vi "log analysis_gps.vi"() -> ()   [LabVIEW 2019] (continued)
76.149993\t101.748821\t8.130800\t-0.795731\t0.628381\t-123.867001\t0.539000\t-0.099000\n\t\n15:49:11.8\tlog_raw\tgps_raw\t#INSPVAXA,USB3,0,49.0,FINESTEERING,2107,283769.800,02000000,471d,15824;INS_ALIGNMENT_COMPLETE,INS_RTKFIXED,37.37104525737,126.72169313095,8.1331,22.3000,-0.3548,-0.2589,0.0390,-0.749813070,0.572311932,213.822472384,0.4366,0.3042,0.5948,0.1140,0.0941,0.0845,0.0971,0.1011,5.0877,0f000001,0*7155f04b\n\tsystem status\tnormal 2 27.800000 0 0\trobot status\t76.002525\t101.557319\t8.133100\t-0.749813\t0.572312\t-123.822472\t0.465000\t0.046000\n\t\n15:49:12.3\tlog_raw\tgps_raw\t#DUALANTENNAHEADINGA,USB3,0,51.5,FINESTEERING,2107,283770.300,02000000,d426,15824;INSUFFICIENT_OBS,NONE,-1.000000000,0.000000000,0.000000000,0.0,0.000000000,0.000000000,\"631T\",11,2,2,2,04,00,20,00*c0be82b5\n\tsystem status\tnormal 2 27.700000 0 0\trobot status\t75.860019\t101.367468\t8.133800\t-0.793741\t0.557880\t-123.760851\t0.448000\t0.089000\n\t\n15:49:12.8\tlog_raw\tgps_raw\t#INSPVAXA,USB3,0,51.5,FINESTEERING,2107,283770.800,02000000,471d,15824;INS_ALIGNMENT_COMPLETE,INS_RTKFIXED,37.37104183450,126.72168993931,8.1368,22.3000,-0.3882,-0.2885,0.0511,-0.819164029,0.307516515,213.418856918,0.4363,0.3032,0.5950,0.1136,0.0937,0.0835,0.0972,0.1011,5.0881,0f000001,0*aed1500e\n\tsystem status\tnormal 2 27.700000 0 0\trobot status\t75.719815\t101.177435\t8.136800\t-0.819164\t0.307517\t-123.418857\t0.470000\t0.060000\n\t\n15:49:13.3\tlog_raw\tgps_raw\t#INSPVAXA,USB3,0,48.5,FINESTEERING,2107,283771.300,02000000,471d,15824;INS_ALIGNMENT_COMPLETE,INS_RTKFIXED,37.37104011891,126.72168833768,8.1396,22.3000,-0.3597,-0.2669,0.0230,-0.734280477,0.363827676,213.144857898,0.4357,0.3026,0.5950,0.1131,0.0936,0.0827,0.0973,0.1011,5.0881,0f000001,0*55c65246\n\tsystem status\tnormal 2 27.700000 0 0\trobot status\t75.577945\t100.987033\t8.139600\t-0.734280\t0.363828\t-123.144858\t0.595000\t-0.151000\n\t\n15:49:13.8\tlog_raw\tgps_raw\t#DUALANTENNAHEADINGA,USB3,0,48.5,FINESTEERING,2107,283771.800,02000000,d426,15824;INSUFFICIENT_OBS,NONE,-1.000000000,0.000000000,0.000000000,0.0,0.000000000,0.000000000,\"631T\",12,2,2,2,04,00,20,00*ba5d6ed0\n\tsystem status\tnormal 2 27.700000 0 0\trobot status\t75.433806\t100.795792\t8.141100\t-0.438126\t0.106263\t-122.855047\t0.459000\t0.049000\n\t\n15:49:14.3\tlog_raw\tgps_raw\t#DUALANTENNAHEADINGA,USB3,0,51.5,FINESTEERING,2107,283772.300,02000000,d426,15824;INSUFFICIENT_OBS,NONE,-1.000000000,0.000000000,0.000000000,0.0,0.000000000,0.000000000,\"631T\",10,2,2,2,04,00,20,00*ccec0b5f\n\tsystem status\tnormal 2 27.800000 0 0\trobot status\t75.294456\t100.606109\t8.143600\t-0.510040\t0.298941\t-122.696971\t0.481000\t0.036000\n\t\n15:49:14.8\tlog_raw\tgps_raw\t#DUALANTENNAHEADINGA,USB3,0,51.5,FINESTEERING,2107,283772.800,02000000,d426,15824;INSUFFICIENT_OBS,NONE,-1.000000000,0.000000000,0.000000000,0.0,0.000000000,0.000000000,\"631T\",11,2,2,2,04,00,20,00*8e3ca933\n\tsystem status\tnormal 2 27.800000 0 0\trobot status\t75.154898\t100.413697\t8.143900\t-0.499119\t0.038857\t-122.482014\t0.607000\t-0.163000\n\t\n15:49:15.3\tlog_raw\tgps_raw\t#DUALANTENNAHEADINGA,USB3,0,51.0,FINESTEERING,2107,283773.300,02000000,d426,15824;INSUFFICIENT_OBS,NONE,-1.000000000,0.000000000,0.000000000,0.0,0.000000000,0.000000000,\"631T\",11,2,2,2,04,00,20,00*23ac6912\n\tsystem status\tnormal 2 27.800000 0 0\trobot status\t75.014278\t100.223479\t8.144500\t-0.192354\t-0.138045\t-122.198268\t0.582000\t-0.140000\n\t\n15:49:15.8\tlog_raw\tgps_raw\t#DUALANTENNAHEADINGA,USB3,0,51.0,FINESTEERING,2107,283773.800,02000000,d426,15824;INSUFFICIENT_OBS,NONE,-1.000000000,0.000000000,0.000000000,0.0,0.000000000,0.000000000,\"631T\",11,2,2,2,04,00,20,00*b69e4b26\n\tsystem status\tnormal 2 27.700000 0 0\trobot status\t74.878118\t100.030778\t8.145700\t-0.513295\t-0.232443\t-122.061694\t0.472000\t0.046000\n\t\n15:49:16.3\tlog_raw\tgps_raw\t#DUALANTENNAHEADINGA,USB3,0,51.5,FINESTEERING,2107,283774.300,02000000,d426,15824;INSUFFICIENT_OBS,NONE,-1.000000000,0.000000000,0.000000000,0.0,0.000000000,0.000000000,\"631T\",10,2,2,2,04,00,20,00*7b4d17c8\n\tsystem status\tnormal 2 27.800000 0 0\trobot status\t74.740846\t99.839920\t8.142500\t-0.454706\t-0.157980\t-121.938744\t0.566000\t-0.113000\n\t\n15:49:16.8\tlog_raw\tgps_raw\t#DUALANTENNAHEADINGA,USB3,0,51.5,FINESTEERING,2107,283774.800,02000000,d426,15824;INSUFFICIENT_OBS,NONE,-1.000000000,0.000000000,0.000000000,0.0,0.000000000,0.000000000,\"631T\",9,2,2,2,04,00,20,00*16022d9f\n\tsystem status\tnormal 2 27.700000 0 0\trobot status\t74.602680\t99.648970\t8.140900\t-0.420847\t-0.146251\t-121.832338\t0.438000\t0.081000\n\t\n15:49:17.3\tlog_raw\tgps_raw\t#INSPVAXA,USB3,0,52.5,FINESTEERING,2107,283775.300,02000000,471d,15824;INS_ALIGNMENT_COMPLETE,INS_RTKFIXED,37.37102638218,126.72167583323,8.1427,22.3000,-0.3501,-0.2557,0.0203,-0.739090378,0.635309618,211.720087902,0.4333,0.3004,0.5913,0.1131,0.0941,0.0802,0.0969,0.1010,5.0876,0f000001,0*37c46ea0\n\tsystem status\tnormal 2 27.800000 0 0\trobot status\t74.470321\t99.462477\t8.142700\t-0.739090\t0.635310\t-121.720088\t0.447000\t0.077000\n\t\n15:49:17.8\tlog_raw\tgps_raw\t#INSPVAXA,USB3,0,52.5,FINESTEERING,2107,283775.800,02000000,471d,15824;INS_ALIGNMENT_COMPLETE,INS_RTKFIXED,37.37102462935,126.72167425219,8.1431,22.3000,-0.3596,-0.2647,0.0054,-0.635685510,0.684071691,211.684016338,0.4333,0.3004,0.5913,0.1131,0.0941,0.0802,0.0969,0.1010,5.0876,0f000001,0*5c9971d0\n\tsystem status\tnormal 2 27.800000 0 0\trobot status\t74.330275\t99.267941\t8.143100\t-0.635686\t0.684072\t-121.684016\t0.576000\t-0.127000\n\t\n15:49:18.3\tlog_raw\tgps_raw\t#DUALANTENNAHEADINGA,USB3,0,52.0,FINESTEERING,2107,283776.300,02000000,d426,15824;INSUFFICIENT_OBS,NONE,-1.000000000,0.000000000,0.000000000,0.0,0.000000000,0.000000000,\"631T\",11,2,2,2,04,00,20,00*8ea80302\n\tsystem status\tnormal 2 27.800000 0 0\trobot status\t74.193470\t99.079089\t8.141100\t-0.450067\t0.650192\t-121.761264\t0.513000\t-0.005000\n\t\n15:49:18.8\tlog_raw\tgps_raw\t#INSPVAXA,USB3,0,52.0,FINESTEERING,2107,283776.800,02000000,471d,15824;INS_ALIGNMENT_COMPLETE,INS_RTKFIXED,37.37102123220,126.72167119947,8.1450,22.3000,-0.3884,-0.2739,0.0352,-0.693294661,0.196719454,211.670955627,0.4336,0.3004,0.5905,0.1143,0.0952,0.0818,0.0967,0.1009,5.0864,0f000001,0*acb72d28\n\tsystem status\tnormal 2 27.800000 0 0\trobot status\t74.059871\t98.890912\t8.145000\t-0.693295\t0.196719\t-121.670956\t0.508000\t-0.007000\n\t\n15:49:19.3\tlog_raw\tgps_raw\t#DUALANTENNAHEADINGA,USB3,0,49.0,FINESTEERING,2107,283777.300,02000000,d426,15824;INSUFFICIENT_OBS,NONE,-1.000000000,0.000000000,0.000000000,0.0,0.000000000,0.000000000,\"631T\",10,2,2,2,04,00,20,00*dd4466ea\n\tsystem status\tnormal 2 27.800000 0 0\trobot status\t73.920832\t98.696227\t8.145400\t-0.727619\t0.204120\t-121.623315\t0.448000\t0.041000\n\t\n15:49:19.8\tlog_raw\tgps_raw\t#INSPVAXA,USB3,0,49.0,FINESTEERING,2107,283777.800,02000000,471d,15824;INS_ALIGNMENT_COMPLETE,INS_RTKFIXED,37.37101775976,126.72166805938,8.1480,22.3000,-0.3623,-0.2643,0.0243,-0.564736999,0.528719086,211.738950079,0.4339,0.3012,0.5898,0.1140,0.0954,0.0814,0.0965,0.1008,5.0862,0f000001,0*673a0e61\n\tsystem status\tnormal 2 27.800000 0 0\trobot status\t73.781727\t98.505527\t8.148000\t-0.564737\t0.528719\t-121.738950\t0.513000\t-0.015000\n\t\n15:49:20.3\tlog_raw\tgps_raw\t#DUALANTENNAHEADINGA,USB3,0,52.0,FINESTEERING,2107,283778.300,02000000,d426,15824;INSUFFICIENT_OBS,NONE,-1.000000000,0.000000000,0.000000000,0.0,0.000000000,0.000000000,\"631T\",10,2,2,2,04,00,20,00*36c9b587\n\tsystem status\tnormal 2 27.800000 0 0\trobot status\t73.643571\t98.311028\t8.150800\t-0.795627\t0.460584\t-121.810377\t0.517000\t-0.009000\n\t\n15:49:20.8\tlog_raw\tgps_raw\t#DUALANTENNAHEADINGA,USB3,0,52.0,FINESTEERING,2107,283778.800,02000000,d426,15824;INSUFFICIENT_OBS,NONE,-1.000000000,0.000000000,0.000000000,0.0,0.000000000,0.000000000,\"631T\",12,2,2,2,04,00,20,00*d74f9142\n\tsystem status\tnormal 2 27.800000 0 0\trobot status\t73.506206\t98.119905\t8.152700\t-0.690272\t0.503378\t-121.737380\t0.499000\t-0.002000\n\t\n15:49:21.3\tlog_raw\tgps_raw\t#DUALANTENNAHEADINGA,USB3,0,51.0,FINESTEERING,2107,283779.300,02000000,d426,15824;INSUFFICIENT_OBS,NONE,-1.000000000,0.000000000,0.000000000,0.0,0.000000000,0.000000000,\"631T\",11,2,2,2,04,00,20,00*203e4aea\n\tsystem status\tnormal 2 27.800000 0 0\trobot status\t73.364976\t97.922589\t8.156700\t-0.651964\t0.039430\t-121.881181\t0.435000\t0.094000\n\t\n15:49:21.8\tlog_raw\tgps_raw\t#DUALANTENNAHEADINGA,USB3,0,51.0,FINESTEERING,2107,283779.800,02000000,d426,15824;INSUFFICIENT_OBS,NONE,-1.000000000,0.000000000,0.000000000,0.0,0.000000000,0.000000000,\"631T\",11,2,2,2,04,00,20,00*b50c68de\n\tsystem status\tnormal 2 27.800000 0 0\trobot status\t73.230256\t97.734889\t8.160800\t-0.719744\t0.364511\t-121.865538\t0.503000\t0.006000\n\t\n15:49:22.3\tlog_raw\tgps_raw\t#DUALANTENNAHEADINGA,USB3,0,51.0,FINESTEERING,2107,283780.300,02000000,d426,15824;INSUFFICIENT_OBS,NONE,-1.000000000,0.000000000,0.000000000,0.0,0.000000000,0.000000000,\"631T\",11,2,2,2,04,00,20,00*92abfb52\n\tsystem status\tnormal 2 27.800000 0 0\trobot status\t73.090819\t97.540360\t8.164900\t-0.527354\t0.221047\t-121.888092\t0.487000\t-0.001000\n\t\n15:49:22.8\tlog_raw\tgps_raw\t#DUALANTENNAHEADINGA,USB3,0,51.0,FINESTEERING,2107,283780.800,02000000,d426,15824;INSUFFICIENT_OBS,NONE,-1.000000000,0.000000000,0.000000000,0.0,0.000000000,0.000000000,\"631T\",13,2,2,2,04,00,20,00*732ddf97\n\tsystem status\tnormal 2 27.800000 0 0\trobot status\t72.956436\t97.348795\t8.168500\t-0.543682\t0.463056\t-121.975660\t0.490000\t-0.003000\n\t\n15:49:23.3\tlog_raw\tgps_raw\t#DUALANTENNAHEADINGA,USB3,0,48.5,FINESTEERING,2107,283781.300,02000000,d426,15824;INSUFFICIENT_OBS,NONE,-1.000000000,0.000000000,0.000000000,0.0,0.000000000,0.000000000,\"631T\",13,2,2,2,04,00,20,00*ffe25397\n\tsystem status\tnormal 2 27.800000 0 0\trobot status\t72.821086\t97.159329\t8.172800\t-0.534217\t0.361937\t-121.905826\t0.581000\t-0.124000\n\t\n15:49:23.8\tlog_raw\tgps_raw\t#DUALANTENNAHEADINGA,USB3,0,48.5,FINESTEERING,2107,283781.800,02000000,d426,15824;INSUFFICIENT_OBS,NONE,-1.000000000,0.000000000,0.000000000,0.0,0.000000000,0.000000000,\"631T\",13,2,2,2,04,00,20,00*6ad071a3\n\tsystem status\tnormal 2 27.800000 0 0\trobot status\t72.686332\t96.969866\t8.178400\t-0.448190\t0.290747\t-121.765545\t0.544000\t-0.090000\n\t\n15:49:24.3\tlog_raw\tgps_raw\t#DUALANTENNAHEADINGA,USB3,0,45.5,FINESTEERING,2107,283782.300,02000000,d426,15824;INSUFFICIENT_OBS,NONE,-1.000000000,0.000000000,0.000000000,0.0,0.000000000,0.000000000,\"631T\",14,2,2,2,04,00,20,00*b956e660\n\tsystem status\tnormal 2 27.800000 0 0\trobot status\t72.547582\t96.775703\t8.181500\t-0.297688\t0.694974\t-121.921446\t0.504000\t0.000000\n\t\n15:49:24.8\tlog_raw\tgps_raw\t#DUALANTENNAHEADINGA,USB3,0,45.5,FINESTEERING,2107,283782.800,02000000,d426,15824;INSUFFICIENT_OBS,NONE,-1.000000000,0.000000000,0.000000000,0.0,0.000000000,0.000000000,\"631T\",15,2,2,2,04,00,20,00*fb86440c\n\tsystem status\tnormal 2 27.800000 0 0\trobot status\t72.415563\t96.590834\t8.185500\t-0.436245\t0.911976\t-121.915066\t0.500000\t0.017000\n\t\n15:49:25.3\tlog_raw\tgps_raw\t#DUALANTENNAHEADINGA,USB3,0,46.5,FINESTEERING,2107,283783.300,02000000,d426,15824;INSUFFICIENT_OBS,NONE,-1.000000000,0.000000000,0.000000000,0.0,0.000000000,0.000000000,\"631T\",14,2,2,2,04,00,20,00*78439955\n\tsystem status\tnormal 2 27.800000 0 0\trobot status\t72.278820\t96.398370\t8.189000\t-0.450895\t0.844522\t-121.900064\t0.493000\t-0.005000\n\t\n15:49:25.8\tlog_raw\tgps_raw\t#DUALANTENNAHEADINGA,USB3,0,46.5,FINESTEERING,2107,283783.800,02000000,d426,15824;INSUFFICIENT_OBS,NONE,-1.000000000,0.000000000,0.000000000,0.0,0.000000000,0.000000000,\"631T\",13,2,2,2,04,00,20,00*a74f302a\n\tsystem status\tnormal 2 27.800000 0 0\trobot status\t72.142409\t96.205979\t8.191200\t-0.508351\t0.608856\t-122.009413\t0.505000\t-0.013000\n\t\n15:49:26.3\tlog_raw\tgps_raw\t#DUALANTENNAHEADINGA,USB3,0,48.5,FINESTEERING,2107,283784.300,02000000,d426,15824;INSUFFICIENT_OBS,NONE,-1.000000000,0.000000000,0.000000000,0.0,0.000000000,0.000000000,\"631T\",12,2,2,2,04,00,20,00*29c9c233\n\tsystem status\tnormal 2 27.800000 0 0\trobot status\t72.005049\t96.015996\t8.197000\t-0.451149\t0.484330\t-122.000685\t0.495000\t0.006000\n\t\n15:49:26.8\tlog_raw\tgps_raw\t#INSPVAXA,USB3,0,48.5,FINESTEERING,2107,283784.850,02000000,471d,15824;INS_ALIGNMENT_COMPLETE,INS_RTKFIXED,37.37099341239,126.72164628694,8.2001,22.3000,-0.3345,-0.2518,0.0438,-0.619275773,0.409325340,212.136895574,0.4352,0.3052,0.5928,0.1145,0.0952,0.0844,0.0964,0.1005,5.0884,0f000001,0*694e34ff\n\tsystem status\tnormal 2 27.800000 0 0\trobot status\t71.853159\t95.803361\t8.200100\t-0.619276\t0.409325\t-122.136896\t0.482000\t-0.002000\n\t\n15:49:27.3\tlog_raw\tgps_raw\t#DUALANTENNAHEADINGA,USB3,0,51.5,FINESTEERING,2107,283785.300,02000000,d426,15824;INSUFFICIENT_OBS,NONE,-1.000000000,0.000000000,0.000000000,0.0,0.000000000,0.000000000,\"631T\",9,2,2,2,04,00,20,00*9cd19b46\n\tsystem status\tnormal 2 27.800000 0 0\trobot status\t71.729501\t95.634009\t8.204000\t-0.435719\t0.399609\t-122.095846\t0.476000\t-0.010000\n\t\n15:49:27.8\tlog_raw\tgps_raw\t#DUALANTENNAHEADINGA,USB3,0,51.5,FINESTEERING,2107,283785.800,02000000,d426,15824;INSUFFICIENT_OBS,NONE,-1.000000000,0.000000000,0.000000000,0.0,0.000000000,0.000000000,\"631T\",10,2,2,2,04,00,20,00*84c8ae0e\n\tsystem status\tnormal 2 27.800000 0 0\trobot status\t71.618681\t95.486877\t8.207900\t-0.336431\t0.419368\t-121.777611\t0.503000\t0.000000\n\t\n15:49:28.3\tlog_raw\tgps_raw\t#DUALANTENNAHEADINGA,USB3,0,51.5,FINESTEERING,2107,283786.300,02000000,d426,15824;INSUFFICIENT_OBS,NONE,-1.000000000,0.000000000,0.000000000,0.0,0.000000000,0.000000000,\"631T\",10,2,2,2,04,00,20,00*a7928151\n\tsystem status\tnormal 2 27.800000 0 0\trobot status\t71.467069\t95.272233\t8.212200\t-0.544144\t0.459789\t-122.100326\t0.513000\t-0.040000\n\t\n15:49:28.8\tlog_raw\tgps_raw\t#DUALANTENNAHEADINGA,USB3,0,51.5,FINESTEERING,2107,283786.800,02000000,d426,15824;INSUFFICIENT_OBS,NONE,-1.000000000,0.000000000,0.000000000,0.0,0.000000000,0.000000000,\"631T\",10,2,2,2,04,00,20,00*32a0a365\n\tsystem status\tnormal 2 27.800000 0 0\trobot status\t71.333321\t95.087329\t8.215100\t-0.468273\t0.209573\t-122.106653\t0.540000\t0.012000\n\t\n15:49:29.3\tlog_raw\tgps_raw\t#DUALANTENNAHEADINGA,USB3,0,51.5,FINESTEERING,2107,283787.300,02000000,d426,15824;INSUFFICIENT_OBS,NONE,-1.000000000,0.000000000,0.000000000,0.0,0.000000000,0.000000000,\"631T\",9,2,2,2,04,00,20,00*9711ff6c\n\tsystem status\tnormal 2 27.800000 0 0\trobot status\t71.195168\t94.900101\t8.218500\t-0.298442\t0.009922\t-122.168983\t0.457000\t-0.007000\n\t\n15:49:29.8\tlog_raw\tgps_raw\t#DUALANTENNAHEADINGA,USB3,0,51.5,FINESTEERING,2107,283787.800,02000000,d426,15824;INSUFFICIENT_OBS,NONE,-1.000000000,0.000000000,0.000000000,0.0,0.000000000,0.000000000,\"631T\",9,2,2,2,04,00,20,00*1a7949a4\n\tsystem status\tnormal 2 27.800000 0 0\trobot status\t71.054623\t94.704881\t8.224300\t-0.425563\t0.019200\t-122.213101\t0.498000\t0.002000\n\t\n15:49:30.3\tlog_raw\tgps_raw\t#DUALANTENNAHEADINGA,USB3,0,51.0,FINESTEERING,2107,283788.300,02000000,d426,15824;INSUFFICIENT_OBS,NONE,-1.000000000,0.000000000,0.000000000,0.0,0.000000000,0.000000000,\"631T\",12,2,2,2,04,00,20,00*e9df57b1\n\tsystem status\tnormal 2 27.800000 0 0\trobot status\t70.919264\t94.520594\t8.227700\t-0.539161\t0.579943\t-122.239809\t0.492000\t0.000000\n\t\n15:49:30.8\tlog_raw\tgps_raw\t#INSPVAXA,USB3,0,51.0,FINESTEERING,2107,283788.850,02000000,471d,15824;INS_ALIGNMENT_COMPLETE,INS_RTKFIXED,37.37097997438,126.72163399809,8.2319,22.3000,-0.3477,-0.2519,0.0287,-0.582557293,0.579304641,212.384981326,0.4350,0.3041,0.5941,0.1138,0.0947,0.0833,0.0968,0.1007,5.0940,0f000001,0*8f3b5f11\n\tsystem status\tnormal 2 27.800000 0 0\trobot status\t70.764633\t94.311958\t8.231900\t-0.582557\t0.579305\t-122.384981\t0.483000\t-0.016000\n\t\n15:49:31.3\tlog_raw\tgps_raw\t#DUALANTENNAHEADINGA,USB3,0,47.5,FINESTEERING,2107,283789.300,02000000,d426,15824;INSUFFICIENT_OBS,NONE,-1.000000000,0.000000000,0.000000000,0.0,0.000000000,0.000000000,\"631T\",11,2,2,2,04,00,20,00*211fe1b3\n\tsystem status\tnormal 2 27.800000 0 0\trobot status\t70.640399\t94.142065\t8.235200\t-0.714458\t0.731325\t-122.445785\t0.500000\t-0.007000\n\t\n15:49:31.8\tlog_raw\tgps_raw\t#DUALANTENNAHEADINGA,USB3,0,47.5,FINESTEERING,2107,283789.800,02000000,d426,15824;INSUFFICIENT_OBS,NONE,-1.000000000,0.000000000,0.000000000,0.0,0.000000000,0.000000000,\"631T\",11,2,2,2,04,00,20,00*b42dc387\n\tsystem status\tnormal 2 27.800000 0 0\trobot status\t70.502929\t93.950748\t8.242200\t-0.958356\t0.812271\t-122.486185\t0.493000\t0.003000\n\t\n15:49:32.3\tlog_raw\tgps_raw\t\tsystem status\tnormal 2 27.800000 0 0\trobot status\t70.364704\t93.763433\t8.246900\t-0.973055\t0.873301\t-122.632437\t0.487000\t-0.013000\n\t\n15:49:32.8\tlog_raw\tgps_raw\t\tsystem status\tnormal 2 27.800000 0 0\trobot status\t70.221231\t93.570837\t8.251300\t-0.845840\t0.736060\t-122.710833\t0.497000\t0.002000\n\t\n15:49:33.3\tlog_raw\tgps_raw\t#DUALANTENNAHEADINGA,USB3,0,48.0,FINESTEERING,2107,283791.300,02000000,d426,15824;INSUFFICIENT_OBS,NONE,-1.000000000,0.000000000,0.000000000,0.0,0.000000000,0.000000000,\"631T\",12,2,2,2,04,00,20,00*82188777\n\tsystem status\tnormal 2 27.800000 0 0\trobot status\t70.080607\t93.379880\t8.255500\t-1.078150\t0.732639\t-122.730012\t0.499000\t0.006000\n\t\n15:49:33.8\tlog_raw\tgps_raw\t#DUALANTENNAHEADINGA,USB3,0,48.0,FINESTEERING,2107,283791.800,02000000,d426,15824;INSUFFICIENT_OBS,NONE,-1.000000000,0.000000000,0.000000000,0.0,0.000000000,0.000000000,\"631T\",11,2,2,2,04,00,20,00*b47c23ea\n\tsystem status\tnormal 2 27.800000 0 0\trobot status\t69.936387\t93.191154\t8.260900\t-0.703435\t0.683274\t-122.771822\t0.499000\t-0.002000\n\t\n15:49:34.3\tlog_raw\tgps_raw\t#DUALANTENNAHEADINGA,USB3,0,50.5,FINESTEERING,2107,283792.300,02000000,d426,15824;INSUFFICIENT_OBS,NONE,-1.000000000,0.000000000,0.000000000,0.0,0.000000000,0.000000000,\"631T\",10,2,2,2,04,00,20,00*50a5f0a4\n\tsystem status\tnormal 2 27.800000 0 0\trobot status\t69.794127\t93.000453\t8.264600\t-0.900507\t0.724571\t-122.856478\t0.489000\t0.001000\n\t\n15:49:34.8\tlog_raw\tgps_raw\t#DUALANTENNAHEADINGA,USB3,0,50.5,FINESTEERING,2107,283792.800,02000000,d426,15824;INSUFFICIENT_OBS,NONE,-1.000000000,0.000000000,0.000000000,0.0,0.000000000,0.000000000,\"631T\",11,2,2,2,04,00,20,00*127552c8\n\tsystem status\tnormal 2 27.800000 0 0\trobot status\t69.649453\t92.812167\t8.268900\t-0.767710\t0.719772\t-122.774208\t0.506000\t0.004000\n\t\n15:49:35.3\tlog_raw\tgps_raw\t#DUALANTENNAHEADINGA,USB3,0,51.0,FINESTEERING,2107,283793.300,02000000,d426,15824;INSUFFICIENT_OBS,NONE,-1.000000000,0.000000000,0.000000000,0.0,0.000000000,0.000000000,\"631T\",12,2,2,2,04,00,20,00*78f7c2e4\n\tsystem status\tnormal 2 27.800000 0 0\trobot status\t69.503579\t92.623917\t8.271900\t-0.646715\t0.260733\t-122.947539\t0.481000\t-0.006000\n\t\n15:49:35.8\tlog_raw\tgps_raw\t#DUALANTENNAHEADINGA,USB3,0,51.0,FINESTEERING,2107,283793.800,02000000,d426,15824;INSUFFICIENT_OBS,NONE,-1.000000000,0.000000000,0.000000000,0.0,0.000000000,0.000000000,\"631T\",12,2,2,2,04,00,20,00*edc5e0d0\n\tsystem status\tnormal 2 27.800000 0 0\trobot status\t69.358793\t92.438468\t8.275400\t-0.583325\t0.396535\t-122.890922\t0.503000\t-0.008000\n\t\n15:49:36.3\tlog_raw\tgps_raw\t#DUALANTENNAHEADINGA,USB3,0,49.0,FINESTEERING,2107,283794.300,02000000,d426,15824;INSUFFICIENT_OBS,NONE,-1.000000000,0.000000000,0.000000000,0.0,0.000000000,0.000000000,\"631T\",12,2,2,2,04,00,20,00*e795402f\n\tsystem status\tnormal 2 27.800000 0 0\trobot status\t69.214021\t92.248222\t8.279000\t-0.756544\t0.479061\t-122.985087\t0.501000\t0.013000\n\t\n15:49:36.8\tlog_raw\tgps_raw\t#INSPVAXA,USB3,0,49.0,FINESTEERING,2107,283794.850,02000000,471d,15824;INS_ALIGNMENT_COMPLETE,INS_RTKFIXED,37.37095950999,126.72161470506,8.2822,22.3000,-0.3469,-0.2852,0.0349,-0.585483256,0.407743515,213.108220245,0.4436,0.3050,0.5933,0.1139,0.0939,0.0807,0.0967,0.1009,5.0986,0f000001,0*2d1ea958\n\tsystem status\tnormal 2 27.800000 0 0\trobot status\t69.055688\t92.040740\t8.282200\t-0.585483\t0.407744\t-123.108220\t0.490000\t-0.009000\n\t\n15:49:37.3\tlog_raw\tgps_raw\t#INSPVAXA,USB3,0,49.5,FINESTEERING,2107,283795.350,02000000,471d,15824;INS_ALIGNMENT_COMPLETE,INS_RTKFIXED,37.37095780554,126.72161308340,8.2866,22.3000,-0.3323,-0.2686,0.0234,-0.679981152,0.368181514,213.212479127,0.4428,0.3050,0.5925,0.1149,0.0952,0.0822,0.0966,0.1008,5.0998,0f000001,0*00d81367\n\tsystem status\tnormal 2 27.800000 0 0\trobot status\t68.912044\t91.851573\t8.286600\t-0.679981\t0.368182\t-123.212479\t0.496000\t0.004000\n\t\n15:49:37.8\tlog_raw\tgps_raw\t#INSPVAXA,USB3,0,49.5,FINESTEERING,2107,283795.850,02000000,471d,15824;INS_ALIGNMENT_COMPLETE,INS_RTKFIXED,37.37095608366,126.72161143693,8.2891,22.3000,-0.3594,-0.2842,0.0245,-0.713487628,0.182586605,213.339171436,0.4428,0.3050,0.5925,0.1149,0.0952,0.0822,0.0966,0.1008,5.0998,0f000001,0*c6ad4823\n\tsystem status\tnormal 2 27.800000 0 0\trobot status\t68.766203\t91.660472\t8.289100\t-0.713488\t0.182587\t-123.339171\t0.498000\t-0.003000\n\t\n15:49:38.3\tlog_raw\tgps_raw\t#DUALANTENNAHEADINGA,USB3,0,49.0,FINESTEERING,2107,283796.300,02000000,d426,15824;INSUFFICIENT_OBS,NONE,-1.000000000,0.000000000,0.000000000,0.0,0.000000000,0.000000000,\"631T\",10,2,2,2,04,00,20,00*48914f6c\n\tsystem status\tnormal 2 27.800000 0 0\trobot status\t68.639733\t91.495855\t8.291100\t-0.637654\t0.495549\t-123.219815\t0.480000\t0.048000\n\t\n15:49:38.8\tlog_raw\tgps_raw\t#DUALANTENNAHEADINGA,USB3,0,49.0,FINESTEERING,2107,283796.800,02000000,d426,15824;INSUFFICIENT_OBS,NONE,-1.000000000,0.000000000,0.000000000,0.0,0.000000000,0.000000000,\"631T\",11,2,2,2,04,00,20,00*0a41ed00\n\tsystem status\tnormal 2 27.800000 0 0\trobot status\t68.496833\t91.305748\t8.293000\t-0.829278\t0.162814\t-123.188565\t0.438000\t0.082000\n\t\n15:49:39.3\tlog_raw\tgps_raw\t#DUALANTENNAHEADINGA,USB3,0,48.0,FINESTEERING,2107,283797.300,02000000,d426,15824;INSUFFICIENT_OBS,NONE,-1.000000000,0.000000000,0.000000000,0.0,0.000000000,0.000000000,\"631T\",9,2,2,2,04,00,20,00*6eb18c36\n\tsystem status\tnormal 2 27.700000 0 0\trobot status\t68.353160\t91.116124\t8.295100\t-0.685896\t0.467526\t-123.151448\t0.470000\t0.044000\n\t\n15:49:39.8\tlog_raw\tgps_raw\t#INSPVAXA,USB3,0,48.0,FINESTEERING,2107,283797.850,02000000,471d,15824;INS_ALIGNMENT_COMPLETE,INS_RTKFIXED,37.37094930309,126.72160503752,8.2955,22.3000,-0.3503,-0.2634,0.0529,-0.883186329,0.520080869,213.088491004,0.4411,0.3046,0.5913,0.1142,0.0943,0.0813,0.0964,0.1007,5.1027,0f000001,0*48f5b9d5\n\tsystem status\tnormal 2 27.700000 0 0\trobot status\t68.199353\t90.907938\t8.295500\t-0.883186\t0.520081\t-123.088491\t0.454000\t0.048000\n\t\n15:49:40.3\tlog_raw\tgps_raw\t#INSPVAXA,USB3,0,49.0,FINESTEERING,2107,283798.350,02000000,471d,15824;INS_ALIGNMENT_COMPLETE,INS_RTKFIXED,37.37094758221,126.72160345161,8.2970,22.3000,-0.3412,-0.2718,0.0078,-0.914982757,0.563532135,212.970746608,0.4404,0.3047,0.5910,0.1139,0.0940,0.0809,0.0964,0.1006,5.1042,0f000001,0*9baeb022\n\tsystem status\tnormal 2 27.700000 0 0\trobot status\t68.058876\t90.716948\t8.297000\t-0.914983\t0.563532\t-122.970747\t0.423000\t0.108000\n\t\n15:49:40.8\tlog_raw\tgps_raw\t#DUALANTENNAHEADINGA,USB3,0,49.0,FINESTEERING,2107,283798.800,02000000,d426,15824;INSUFFICIENT_OBS,NONE,-1.000000000,0.000000000,0.000000000,0.0,0.000000000,0.000000000,\"631T\",12,2,2,2,04,00,20,00*c6945d74\n\tsystem status\tnormal 2 27.700000 0 0\trobot status\t67.933675\t90.545256\t8.298900\t-1.010475\t0.600709\t-122.903426\t0.483000\t0.041000\n\t\n15:49:41.3\tlog_raw\tgps_raw\t#DUALANTENNAHEADINGA,USB3,0,45.5,FINESTEERING,2107,283799.300,02000000,d426,15824;INSUFFICIENT_OBS,NONE,-1.000000000,0.000000000,0.000000000,0.0,0.000000000,0.000000000,\"631T\",11,2,2,2,04,00,20,00*16f4fe8f\n\tsystem status\tnormal 2 27.700000 0 0\trobot status\t67.793618\t90.353471\t8.299900\t-0.899840\t0.265209\t-122.789147\t0.422000\t0.082000\n\t\n15:49:41.8\tlog_raw\tgps_raw\t\tsystem status\tnormal 2 27.700000 0 0\trobot status\t67.676243\t90.195928\t8.301100\t-0.734435\t0.501413\t-122.556999\t0.511000\t0.000000\n\t\n15:49:42.3\tlog_raw\tgps_raw\t#INSPVAXA,USB3,0,49.0,FINESTEERING,2107,283800.350,02000000,471d,15824;INS_ALIGNMENT_COMPLETE,INS_RTKFIXED,37.37094091423,126.72159737065,8.3045,22.3000,-0.3067,-0.2479,0.0203,-0.819842443,0.191371077,212.561808426,0.4393,0.3042,0.5904,0.1136,0.0943,0.0803,0.0963,0.1005,5.1071,0f000001,0*87713df7\n\tsystem status\tnormal 2 27.800000 0 0\trobot status\t67.520235\t89.976909\t8.304500\t-0.819842\t0.191371\t-122.561808\t0.545000\t-0.122000\n\t\n15:49:42.8\tlog_raw\tgps_raw\t#INSPVAXA,USB3,0,49.0,FINESTEERING,2107,283800.850,02000000,471d,15824;INS_ALIGNMENT_COMPLETE,INS_RTKFIXED,37.37093917106,126.72159578711,8.3082,22.3000,-0.3234,-0.2591,0.0222,-0.646837907,0.336367436,212.664833979,0.4393,0.3042,0.5904,0.1136,0.0943,0.0803,0.0963,0.1005,5.1071,0f000001,0*a47e26e8\n\tsystem status\tnormal 2 27.800000 0 0\trobot status\t67.379967\t89.783445\t8.308200\t-0.646838\t0.336367\t-122.664834\t0.433000\t0.090000\n\t\n15:49:43.3\tlog_raw\tgps_raw\t#INSPVAXA,USB3,0,42.0,FINESTEERING,2107,283801.350,02000000,471d,15824;INS_ALIGNMENT_COMPLETE,INS_RTKFIXED,37.37093749345,126.72159425291,8.3098,22.3000,-0.3764,-0.2836,0.0471,-0.642147741,0.485055187,212.666460459,0.4391,0.3035,0.5903,0.1145,0.0947,0.0815,0.0963,0.1005,5.1074,0f000001,0*cfb387f2\n\tsystem status\tnormal 2 27.800000 0 0\trobot status\t67.244070\t89.597257\t8.309800\t-0.642148\t0.485055\t-122.666460\t0.517000\t-0.018000\n\t\n15:49:43.8\tlog_raw\tgps_raw\t#INSPVAXA,USB3,0,42.0,FINESTEERING,2107,283801.850,02000000,471d,15824;INS_ALIGNMENT_COMPLETE,INS_RTKFIXED,37.37093581786,126.72159270156,8.3102,22.3000,-0.3221,-0.2542,0.0038,-0.637890069,0.520458025,212.703870431,0.4391,0.3035,0.5903,0.1145,0.0947,0.0815,0.0963,0.1005,5.1074,0f000001,0*42dc58c1\n\tsystem status\tnormal 2 27.800000 0 0\trobot status\t67.106654\t89.411294\t8.310200\t-0.637890\t0.520458\t-122.703870\t0.478000\t0.000000\n\t\n15:49:44.3\tlog_raw\tgps_raw\t#INSPVAXA,USB3,0,48.0,FINESTEERING,2107,283802.350,02000000,471d,15824;INS_ALIGNMENT_COMPLETE,INS_RTKFIXED,37.37093409830,126.72159111901,8.3142,22.3000,-0.3534,-0.2655,0.0351,-0.709498391,0.532234116,212.787033062,0.4389,0.3043,0.5904,0.1141,0.0944,0.0812,0.0962,0.1004,5.1086,0f000001,0*ada231a9\n\tsystem status\tnormal 2 27.700000 0 0\trobot status\t66.966475\t89.220450\t8.314200\t-0.709498\t0.532234\t-122.787033\t0.488000\t-0.004000\n\t\n15:49:44.8\tlog_raw\tgps_raw\t#INSPVAXA,USB3,0,48.0,FINESTEERING,2107,283802.850,02000000,471d,15824;INS_ALIGNMENT_COMPLETE,INS_RTKFIXED,37.37093238773,126.72158954092,8.3176,22.3000,-0.3340,-0.2726,0.0399,-0.642602467,0.406541705,212.810181353,0.4389,0.3043,0.5904,0.1141,0.0944,0.0812,0.0962,0.1004,5.1086,0f000001,0*fb1d3214\n\tsystem status\tnormal 2 27.800000 0 0\trobot status\t66.826690\t89.030604\t8.317600\t-0.642602\t0.406542\t-122.810181\t0.481000\t-0.002000\n\t\n15:49:45.3\tlog_raw\tgps_raw\t#INSPVAXA,USB3,0,50.0,FINESTEERING,2107,283803.350,02000000,471d,15824;INS_ALIGNMENT_COMPLETE,INS_RTKFIXED,37.37093069995,126.72158798195,8.3220,22.3000,-0.3417,-0.2608,0.0173,-0.694649524,0.610927882,212.865796142,0.4386,0.3050,0.5904,0.1147,0.0949,0.0821,0.0962,0.1004,5.1101,0f000001,0*664f4704\n\tsystem status\tnormal 2 27.800000 0 0\trobot status\t66.688599\t88.843288\t8.322000\t-0.694650\t0.610928\t-122.865796\t0.491000\t-0.004000\n\t\n15:49:45.8\tlog_raw\tgps_raw\t#INSPVAXA,USB3,0,50.0,FINESTEERING,2107,283803.850,02000000,471d,15824;INS_ALIGNMENT_COMPLETE,INS_RTKFIXED,37.37092900254,126.72158638121,8.3251,22.3000,-0.3538,-0.2865,0.0254,-0.433488286,0.440900980,212.995869774,0.4386,0.3050,0.5904,0.1147,0.0949,0.0821,0.0962,0.1004,5.1101,0f000001,0*a84e9ea6\n\tsystem status\tnormal 2 27.800000 0 0\trobot status\t66.546808\t88.654903\t8.325100\t-0.433488\t0.440901\t-122.995870\t0.505000\t-0.016000\n\t\n15:49:46.3\tlog_raw\tgps_raw\t#INSPVAXA,USB3,0,48.0,FINESTEERING,2107,283804.350,02000000,471d,15824;INS_ALIGNMENT_COMPLETE,INS_RTKFIXED,37.37092729858,126.72158475162,8.3262,22.3000,-0.3346,-0.2736,0.0337,-0.198500988,0.485164152,213.066525624,0.4382,0.3051,0.5905,0.1141,0.0944,0.0817,0.0962,0.1004,5.1114,0f000001,0*c4e8da54\n\tsystem status\tnormal 2 27.800000 0 0\trobot status\t66.402462\t88.465790\t8.326200\t-0.198501\t0.485164\t-123.066526\t0.483000\t-0.010000\n\t\n15:49:46.8\tlog_raw\tgps_raw\t#INSPVAXA,USB3,0,48.0,FINESTEERING,2107,283804.850,02000000,471d,15824;INS_ALIGNMENT_COMPLETE,INS_RTKFIXED,37.37092559356,126.72158315411,8.3286,22.3000,-0.3344,-0.2698,0.0356,-0.560548188,0.428951869,213.152040125,0.4382,0.3051,0.5905,0.1141,0.0944,0.0817,0.0962,0.1004,5.1114,0f000001,0*865f3348\n\tsystem status\tnormal 2 27.800000 0 0\trobot status\t66.260957\t88.276561\t8.328600\t-0.560548\t0.428952\t-123.152040\t0.512000\t0.002000\n\t\n15:49:47.3\tlog_raw\tgps_raw\t#INSPVAXA,USB3,0,50.5,FINESTEERING,2107,283805.350,02000000,471d,15824;INS_ALIGNMENT_COMPLETE,INS_RTKFIXED,37.37092390925,126.72158151800,8.3310,22.3000,-0.3577,-0.2766,0.0312,-0.244742363,0.378624826,213.232619206,0.4377,0.3050,0.5905,0.1137,0.0939,0.0814,0.0962,0.1003,5.1129,0f000001,0*93a69a58\n\tsystem status\tnormal 2 27.800000 0 0\trobot status\t66.116033\t88.089629\t8.331000\t-0.244742\t0.378625\t-123.232619\t0.499000\t-0.009000\n\t\n15:49:47.8\tlog_raw\tgps_raw\t\tsystem status\tnormal 2 27.800000 0 0\trobot status\t65.986520\t87.922956\t8.333200\t-0.008516\t0.673932\t-123.197581\t0.482000\t0.005000\n\t\n15:49:48.3\tlog_raw\tgps_raw\t#INSPVAXA,USB3,0,51.0,FINESTEERING,2107,283806.350,02000000,471d,15824;INS_ALIGNMENT_COMPLETE,INS_RTKFIXED,37.37092052937,126.72157829690,8.3375,22.3000,-0.3440,-0.2795,0.0245,-0.465963804,0.886312303,213.254279307,0.4369,0.3047,0.5904,0.1133,0.0936,0.0810,0.0962,0.1003,5.1143,0f000001,0*ac9069ee\n\tsystem status\tnormal 2 27.800000 0 0\trobot status\t65.830713\t87.714517\t8.337500\t-0.465964\t0.886312\t-123.254279\t0.502000\t0.001000\n\t\n15:49:48.8\tlog_raw\tgps_raw\t#INSPVAXA,USB3,0,51.0,FINESTEERING,2107,283806.850,02000000,471d,15824;INS_ALIGNMENT_COMPLETE,INS_RTKFIXED,37.37091879437,126.72157664668,8.3407,22.3000,-0.3462,-0.2861,0.0240,-0.657037721,0.825600095,213.429652251,0.4369,0.3047,0.5904,0.1133,0.0936,0.0810,0.0962,0.1003,5.1143,0f000001,0*17c14289\n\tsystem status\tnormal 2 27.800000 0 0\trobot status\t65.684539\t87.521960\t8.340700\t-0.657038\t0.825600\t-123.429652\t0.499000\t-0.003000\n\t\n15:49:49.3\tlog_raw\tgps_raw\t\tsystem status\tnormal 2 27.800000 0 0\trobot status\t65.554303\t87.354683\t8.344900\t-0.435824\t0.698200\t-123.493110\t0.489000\t-0.010000\n\t\n15:49:49.8\tlog_raw\tgps_raw\t#INSPVAXA,USB3,0,48.5,FINESTEERING,2107,283807.850,02000000,471d,15824;INS_ALIGNMENT_COMPLETE,INS_RTKFIXED,37.37091541659,126.72157338154,8.3525,22.3000,-0.3441,-0.2744,0.0198,-0.559398750,0.972716137,213.514077628,0.4363,0.3044,0.5901,0.1131,0.0934,0.0806,0.0963,0.1003,5.1156,0f000001,0*75ff1fc6\n\tsystem status\tnormal 2 27.800000 0 0\trobot status\t65.395319\t87.147080\t8.352500\t-0.559399\t0.972716\t-123.514078\t0.504000\t0.008000\n\t\n15:49:50.3\tlog_raw\tgps_raw\t#INSPVAXA,USB3,0,44.5,FINESTEERING,2107,283808.350,02000000,471d,15824;INS_ALIGNMENT_COMPLETE,INS_RTKFIXED,37.37091372939,126.72157175918,8.3549,22.3000,-0.3553,-0.2831,0.0286,-0.709577121,1.164612328,213.658250013,0.4360,0.3038,0.5897,0.1132,0.0934,0.0803,0.0963,0.1003,5.1169,0f000001,0*14793968\n\tsystem status\tnormal 2 27.800000 0 0\trobot status\t65.251613\t86.959828\t8.354900\t-0.709577\t1.164612\t-123.658250\t0.503000\t-0.012000\n\t\n15:49:50.8\tlog_raw\tgps_raw\t#INSPVAXA,USB3,0,44.5,FINESTEERING,2107,283808.850,02000000,471d,15824;INS_ALIGNMENT_COMPLETE,INS_RTKFIXED,37.37091204717,126.72157012311,8.3593,22.3000,-0.3351,-0.2933,0.0335,-0.548646333,0.899552178,213.508678338,0.4360,0.3038,0.5897,0.1132,0.0934,0.0803,0.0963,0.1003,5.1169,0f000001,0*e79048d5\n\tsystem status\tnormal 2 27.800000 0 0\trobot status\t65.106692\t86.773129\t8.359300\t-0.548646\t0.899552\t-123.508678\t0.480000\t0.004000\n\t\n15:49:51.3\tlog_raw\tgps_raw\t#INSPVAXA,USB3,0,46.0,FINESTEERING,2107,283809.350,02000000,471d,15824;INS_ALIGNMENT_COMPLETE,INS_RTKFIXED,37.37091031450,126.72156845279,8.3650,22.3000,-0.3479,-0.2887,0.0292,-0.530979071,0.488041271,213.615691599,0.4360,0.3037,0.5892,0.1129,0.0933,0.0800,0.0963,0.1003,5.1177,0f000001,0*4685a971\n\tsystem status\tnormal 2 27.800000 0 0\trobot status\t64.958738\t86.580830\t8.365000\t-0.530979\t0.488041\t-123.615692\t0.500000\t0.006000\n\t\n15:49:51.8\tlog_raw\tgps_raw\t#INSPVAXA,USB3,0,46.0,FINESTEERING,2107,283809.850,02000000,471d,15824;INS_ALIGNMENT_COMPLETE,INS_RTKFIXED,37.37090862475,126.72156681870,8.3704,22.3000,-0.3507,-0.2732,0.0187,-0.627436643,0.484815097,213.766429758,0.4360,0.3037,0.5892,0.1129,0.0933,0.0800,0.0963,0.1003,5.1177,0f000001,0*042f58f5\n\tsystem status\tnormal 2 27.800000 0 0\trobot status\t64.813993\t86.393295\t8.370400\t-0.627437\t0.484815\t-123.766430\t0.498000\t-0.012000\n\t\n15:49:52.3\tlog_raw\tgps_raw\t#INSPVAXA,USB3,0,46.5,FINESTEERING,2107,283810.350,02000000,471d,15824;INS_ALIGNMENT_COMPLETE,INS_RTKFIXED,37.37090694651,126.72156520391,8.3753,22.3000,-0.3165,-0.2719,0.0394,-0.596255769,0.780970899,213.702239240,0.4358,0.3031,0.5888,0.1129,0.0933,0.0798,0.0963,0.1003,5.1187,0f000001,0*196b83f4\n\tsystem status\tnormal 2 27.800000 0 0\trobot status\t64.670957\t86.207038\t8.375300\t-0.596256\t0.780971\t-123.702239\t0.428000\t0.086000\n\t\n15:49:52.8\tlog_raw\tgps_raw\t#INSPVAXA,USB3,0,46.5,FINESTEERING,2107,283810.850,02000000,471d,15824;INS_ALIGNMENT_COMPLETE,INS_RTKFIXED,37.37090525382,126.72156361193,8.3794,22.3000,-0.3598,-0.2713,0.0249,-0.973711193,1.074767761,213.656129114,0.4358,0.3031,0.5888,0.1129,0.0933,0.0798,0.0963,0.1003,5.1187,0f000001,0*60ffddbf\n\tsystem status\tnormal 2 27.700000 0 0\trobot status\t64.529943\t86.019176\t8.379400\t-0.973711\t1.074768\t-123.656129\t0.602000\t-0.133000\n\t\n15:49:53.3\tlog_raw\tgps_raw\t#INSPVAXA,USB3,0,49.0,FINESTEERING,2107,283811.350,02000000,471d,15824;INS_ALIGNMENT_COMPLETE,INS_RTKFIXED,37.37090357920,126.72156200390,8.3845,22.3000,-0.3442,-0.2800,0.0256,-0.979609219,0.857511693,213.501334190,0.4355,0.3025,0.5885,0.1131,0.0935,0.0796,0.0962,0.1002,5.1194,0f000001,0*aa11bf3c\n\tsystem status\tnormal 2 27.700000 0 0\trobot status\t64.387506\t85.833320\t8.384500\t-0.979609\t0.857512\t-123.501334\t0.560000\t-0.119000\n\t\n15:49:53.8\tlog_raw\tgps_raw\t#INSPVAXA,USB3,0,49.0,FINESTEERING,2107,283811.850,02000000,471d,15824;INS_ALIGNMENT_COMPLETE,INS_RTKFIXED,37.37090187370,126.72156034536,8.3910,22.3000,-0.3251,-0.2819,0.0474,-0.722859580,0.747515698,213.305789576,0.4355,0.3025,0.5885,0.1131,0.0935,0.0796,0.0962,0.1002,5.1194,0f000001,0*3fd13bdf\n\tsystem status\tnormal 2 27.800000 0 0\trobot status\t64.240595\t85.644037\t8.391000\t-0.722860\t0.747516\t-123.305790\t0.574000\t-0.130000\n\t\n15:49:54.3\tlog_raw\tgps_raw\t#INSPVAXA,USB3,0,49.5,FINESTEERING,2107,283812.350,02000000,471d,15824;INS_ALIGNMENT_COMPLETE,INS_RTKFIXED,37.37090016195,126.72155872579,8.3941,22.3000,-0.3301,-0.2714,0.0230,-0.816861765,0.807045897,213.365991854,0.4358,0.3019,0.5880,0.1129,0.0935,0.0794,0.0962,0.1002,5.1192,0f000001,0*4c65b004\n\tsystem status\tnormal 2 27.800000 0 0\trobot status\t64.097136\t85.454060\t8.394100\t-0.816862\t0.807046\t-123.365992\t0.437000\t0.092000\n\t\n15:49:54.8\tlog_raw\tgps_raw\t#INSPVAXA,USB3,0,49.5,FINESTEERING,2107,283812.850,02000000,471d,15824;INS_ALIGNMENT_COMPLETE,INS_RTKFIXED,37.37089850948,126.72155716436,8.4007,22.3000,-0.3466,-0.2674,0.0245,-1.010459105,1.203472326,213.239594675,0.4358,0.3019,0.5880,0.1129,0.0935,0.0794,0.0962,0.1002,5.1192,0f000001,0*1434da4d\n\tsystem status\tnormal 2 27.700000 0 0\trobot status\t63.958827\t85.270663\t8.400700\t-1.010459\t1.203472\t-123.239595\t0.598000\t-0.162000\n\t\n15:49:55.3\tlog_raw\tgps_raw\t#INSPVAXA,USB3,0,49.0,FINESTEERING,2107,283813.350,02000000,471d,15824;INS_ALIGNMENT_COMPLETE,INS_RTKFIXED,37.37089680632,126.72155557603,8.4063,22.3000,-0.3291,-0.2810,0.0480,-0.955572188,1.123844377,213.096084553,0.4352,0.3013,0.5874,0.1129,0.0933,0.0793,0.0961,0.1001,5.1186,0f000001,0*817699e2\n\tsystem status\tnormal 2 27.700000 0 0\trobot status\t63.818136\t85.081639\t8.406300\t-0.955572\t1.123844\t-123.096085\t0.440000\t0.089000\n\t\n15:49:55.8\tlog_raw\tgps_raw\t#INSPVAXA,USB3,0,49.0,FINESTEERING,2107,283813.850,02000000,471d,15824;INS_ALIGNMENT_COMPLETE,INS_RTKFIXED,37.37089510360,126.72155399997,8.4119,22.3000,-0.3389,-0.2720,0.0269,-0.936574530,0.986776176,213.030169664,0.4352,0.3013,0.5874,0.1129,0.0933,0.0793,0.0961,0.1001,5.1186,0f000001,0*5c3995b3\n\tsystem status\tnormal 2 27.700000 0 0\trobot status\t63.678531\t84.892664\t8.411900\t-0.936575\t0.986776\t-123.030170\t0.431000\t0.096000\n\t\n15:49:56.3\tlog_raw\tgps_raw\t#INSPVAXA,USB3,0,49.5,FINESTEERING,2107,283814.350,02000000,471d,15824;INS_ALIGNMENT_COMPLETE,INS_RTKFIXED,37.37089337891,126.72155240702,8.4168,22.3000,-0.3379,-0.2725,0.0259,-0.990897752,0.543543172,212.990799562,0.4348,0.3013,0.5869,0.1127,0.0935,0.0792,0.0960,0.1000,5.1178,0f000001,0*80d17f12\n\tsystem status\tnormal 2 27.800000 0 0\trobot status\t63.537430\t84.701251\t8.416800\t-0.990898\t0.543543\t-122.990800\t0.444000\t0.071000\n\t\n15:49:56.8\tlog_raw\tgps_raw\t\tsystem status\tnormal 2 27.700000 0 0\trobot status\t63.399172\t84.512548\t8.420400\t-1.050118\t0.471957\t-122.840638\t0.484000\t0.039000\n\t\n15:49:57.3\tlog_raw\tgps_raw\t#INSPVAXA,USB3,0,49.0,FINESTEERING,2107,283815.350,02000000,471d,15824;INS_ALIGNMENT_COMPLETE,INS_RTKFIXED,37.37088996706,126.72154929258,8.4245,22.3000,-0.3434,-0.2641,0.0250,-1.164432895,0.561258596,212.864234070,0.4342,0.3009,0.5863,0.1129,0.0938,0.0795,0.0959,0.1000,5.1167,0f000001,0*c7d2a868\n\tsystem status\tnormal 2 27.800000 0 0\trobot status\t63.261558\t84.322591\t8.424500\t-1.164433\t0.561259\t-122.864234\t0.465000\t0.034000\n\t\n15:49:57.8\tlog_raw\tgps_raw\t#INSPVAXA,USB3,0,49.0,FINESTEERING,2107,283815.850,02000000,471d,15824;INS_ALIGNMENT_COMPLETE,INS_RTKFIXED,37.37088825034,126.72154772822,8.4276,22.3000,-0.3370,-0.2619,0.0268,-1.087119592,0.609799872,212.870793479,0.4342,0.3009,0.5863,0.1129,0.0938,0.0795,0.0959,0.1000,5.1167,0f000001,0*f57586d5\n\tsystem status\tnormal 2 27.800000 0 0\trobot status\t63.122989\t84.132062\t8.427600\t-1.087120\t0.609800\t-122.870793\t0.461000\t0.024000\n\t\n15:49:58.3\tlog_raw\tgps_raw\t#INSPVAXA,USB3,0,45.5,FINESTEERING,2107,283816.350,02000000,471d,15824;INS_ALIGNMENT_COMPLETE,INS_RTKFIXED,37.37088648339,126.72154610950,8.4307,22.3000,-0.3394,-0.2623,0.0227,-0.831042768,0.509272652,212.987067657,0.4339,0.3006,0.5859,0.1127,0.0936,0.0794,0.0958,0.0999,5.1151,0f000001,0*c540a699\n\tsystem status\tnormal 2 27.800000 0 0\trobot status\t62.979606\t83.935959\t8.430700\t-0.831043\t0.509273\t-122.987068\t0.502000\t-0.011000\n\t\n15:49:58.8\tlog_raw\tgps_raw\t#INSPVAXA,USB3,0,45.5,FINESTEERING,2107,283816.850,02000000,471d,15824;INS_ALIGNMENT_COMPLETE,INS_RTKFIXED,37.37088478874,126.72154457975,8.4339,22.3000,-0.3715,-0.2876,0.0149,-0.938105772,0.365449923,213.063297584,0.4339,0.3006,0.5859,0.1127,0.0936,0.0794,0.0958,0.0999,5.1151,0f000001,0*840abd00\n\tsystem status\tnormal 2 27.800000 0 0\trobot status\t62.844103\t83.747880\t8.433900\t-0.938106\t0.365450\t-123.063298\t0.513000\t-0.009000\n\t\n15:49:59.3\tlog_raw\tgps_raw\t#INSPVAXA,USB3,0,46.5,FINESTEERING,2107,283817.350,02000000,471d,15824;INS_ALIGNMENT_COMPLETE,INS_RTKFIXED,37.37088307773,126.72154302879,8.4374,22.3000,-0.3594,-0.2773,0.0287,-0.958522380,0.243905829,212.991264938,0.4341,0.3007,0.5858,0.1132,0.0942,0.0801,0.0958,0.0999,5.1140,0f000001,0*fa6ad0ef\n\tsystem status\tnormal 2 27.800000 0 0\trobot status\t62.706722\t83.557985\t8.437400\t-0.958522\t0.243906\t-122.991265\t0.453000\t0.045000\n\t\n15:49:59.8\tlog_raw\tgps_raw\t#INSPVAXA,USB3,0,46.5,FINESTEERING,2107,283817.850,02000000,471d,15824;
